vi "autoRelativeToAbsolute.vi"(10 "command in":string[](array[string]), 11 "datas":T1) -> (3 "adjusted command":string[](array[string]))   [LabVIEW 2012]
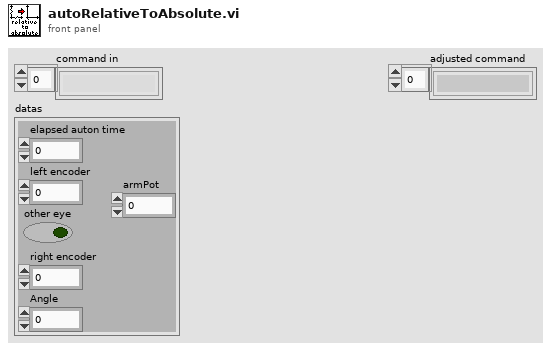
[diagram p1: front panel]
types:
  T1 = cluster{"elapsed auton time":dbl, "left encoder":dbl, "other eye":bool, "right encoder":dbl, "Angle":dbl, "armPot":dbl}
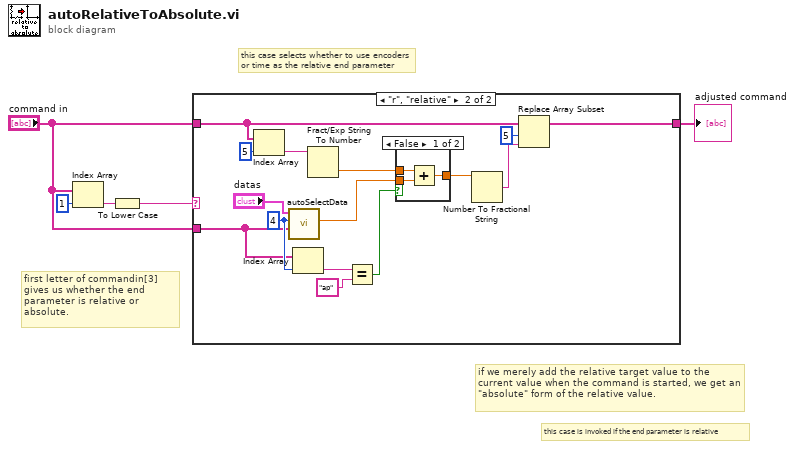
[diagram p0: block diagram]
diagram:
  # "this case is invoked if the end parameter is relative"
  # "if we merely add the relative target value to the current value when the command is started, we get an \"absolute\" form of the relative value."
  # "this case selects whether to use encoders or time as the relative end parameter"
  # "first letter of commandin[3] gives us whether the end parameter is relative or absolute."
  n1 = Index Array(array="command in", index=1) -> (element=w2:string)
  n2 = To Lower Case(string=w2) -> (all lower case string=w1:string)
  n3 = case shown="\"r\", \"relative\"" w1 {
    tunnel: "command in" -> [w6 w18]
    tunnel: [w6 w17] -> w4
    tunnel: "command in" -> [_ w10]
    frame "a", "absolute", Default {
      # "absolute values.  Do nothing."
    }
    frame "r", "relative" {
      w12 = u8 4 ("index")
      n4 = Index Array(array=w18, index=5) -> (element=w20:string)
      n5 = call "autoSelectData.vi"("command and parameters in"=w10, "index"=w12, "sensor datas"="datas") -> ("accessed value"=w14:dbl)  [unwired: 8 in]
      n6 = Index Array(array=w10, index=w12) -> (element=w9:string)
      n7 = Fract/Exp String To Number(string=w20) -> (number=w19:dbl)  [unwired: 3 in, 1 out]
      n8 = Equal?(x=w9, y="ap") -> (x = y?=w7:bool)
      n9 = case shown="False" w7 {
        tunnel: w19 -> [w24 w25]
        tunnel: w14 -> [w23 _]
        tunnel: [w22 w25] -> w13
        frame False {
          n10 = Add(x=w24, y=w23) -> (x+y=w22:dbl)
        }
        frame True {
        }
      }
      n11 = Number To Fractional String(number=w13) -> (F-format string=w15:string)  [unwired: 3 in]
      n12 = Replace Array Subset(array=w18, new element=w15, index=5) -> (w17:string[])
    }
  }
  "adjusted command" <- w4
